vi "FlowRateReadout.vi"(3 "error in":errorcluster, 4 "LC2 Pin":i32, 5 "LC1 Pin":i32, 6 "Handle In":i32) -> (0 "error out":errorcluster[](array[cluster]), 1 "LS2 Voltage Reading":dbl format="%.6f", 2 "LS1 Voltage Reading":dbl format="%.6f")   [LabVIEW 2021]
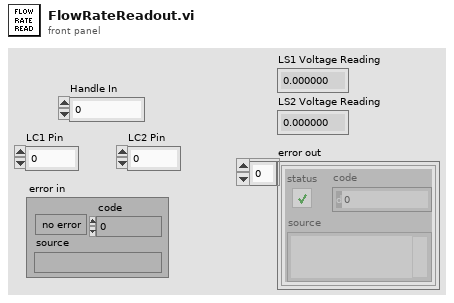
[diagram p1: front panel]
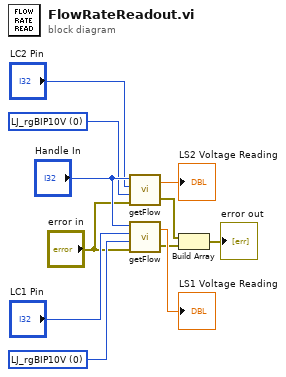
[diagram p0: block diagram]
diagram:
  w7 = u16 0 items=["LJ_rgBIP10V", "LJ_rgBIP1V", "LJ_rgBIPP1V", "LJ_rgBIPP01V"] ("AIN Range")
  w8 = u16 0 items=["LJ_rgBIP10V", "LJ_rgBIP1V", "LJ_rgBIPP1V", "LJ_rgBIPP01V"] ("AIN Range")
  n1 = call "getFlow.vi"("error in"="error in", "AIN Range"=w7, "+ Channel"="LC2 Pin", "Handle In"="Handle In") -> ("error out"=w3:errorcluster, "Voltage Reading"=→"LS2 Voltage Reading":dbl)
  n2 = call "getFlow.vi"("error in"="error in", "AIN Range"=w8, "+ Channel"="LC1 Pin", "Handle In"="Handle In") -> ("error out"=w2:errorcluster, "Voltage Reading"=→"LS1 Voltage Reading":dbl)
  n3 = Build Array(w3, w2) -> (→"error out":errorcluster[])
